vi "InitBrd.vi"(0 "xckdly":u32 format="%.0x", 4 "pixel":u32=5400, 5 "flag816":u32=1) -> ()   [LabVIEW 2015]
uses:
  board.vis/ESLSCDLL.dll
panel:
  in  "pclk":u32 format="%.0x"
  # "set read frequency"
  # "8bit=2/12-16bit=1"
  # "not used"
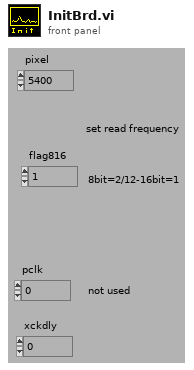
[diagram p1: front panel]
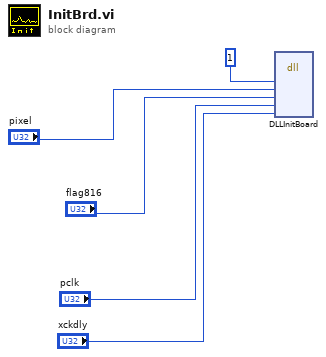
[diagram p0: block diagram]
diagram:
  n1 = dll-call lib="C:/ENTW/PCIE/64bit/lv64/lv64_eventdriven/board.vis/ESLSCDLL.dll" fn="DLLInitBoard"("drv"=u32 1, "pixel"="pixel", "flag816"="flag816", "pclk"="pclk", "xckdelay"="xckdly") -> ()  [unwired: 9 in, 2 out]
